vi "visa_write.vi"() -> ()   [LabVIEW 2016]
uses:
  <vilib>/Instr/_visa.llb/VISA Configure Serial Port (Instr).vi
panel:
  in  "停止":bool
  out "写入缓冲区":string
  out "输出数组":i32[](array[numeric])
  in  "目标位置":i32[](array[numeric])
  in  "当前位置":i32[](array[numeric])
  in  "串口配置":T1={"波特率"=115200, "奇偶校验位"=0, "停止位"=10, "流控制"=0, "数据位"=8} {"数据位" items=["8"=8]; "流控制" items=["无"=0, "XON/XOFF"=1, "RTS/CTS"=2, "DTR/DSR"=4]; "停止位" items=["1.0"=10, "2.0"=15, "3.0"=20]; "奇偶校验位" items=["None"]; "波特率" items=["115200"=115200]}
  in  "VISA资源名称":refnum<visa-resource-name>
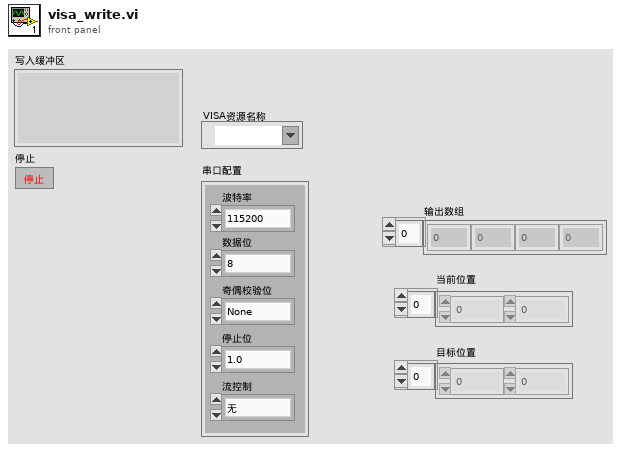
[diagram p1: front panel]
types:
  T1 = cluster{"波特率":u32, "奇偶校验位":u16, "停止位":u16, "流控制":u16, "数据位":u32}
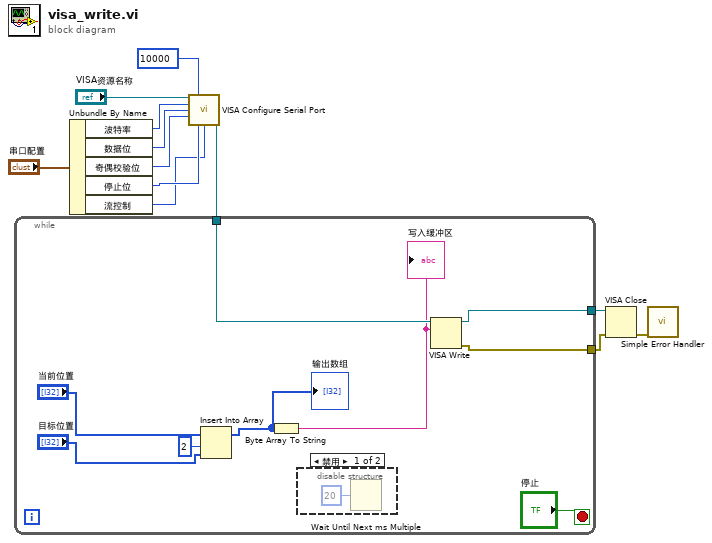
[diagram p0: block diagram]
diagram:
  n1 = Unbundle By Name("串口配置") -> ("波特率"=w10:u32, "数据位"=w9:u32, "奇偶校验位"=w8:u16, "停止位"=w7:u16, "流控制"=w6:u16)
  n2 = call-poly "VISA Configure Serial Port"("VISA resource name"="VISA资源名称", "timeout (10sec)"=u32 10000, "baud rate (9600)"=w10, "data bits (8)"=w9, "parity (0:none)"=w8, "stop bits (10: 1 bit)"=w7, "flow control (0:none)"=w6) -> ("VISA resource name out"=w5:refnum<visa-resource-name>)  [unwired: 7 in, 1 out]
  n3 = while {
    tunnel: w5 -> [w21]
    tunnel: [w14] -> w2
    tunnel: [w13] -> w1
    stop <- "停止" stop-if-true
    n4 = Insert Into Array(array="当前位置", index=2 ("索引"), new element="目标位置") -> (w15:i32[])
    "输出数组" <- w15
    n5 = Byte Array To String ("字节数组至字符串转换")(unsigned byte array=w15) -> (string=w20:string)
    "写入缓冲区" <- w20
    n6 = disable-structure shown="禁用" {
      frame Disabled {
        n7 = Wait Until Next ms Multiple(millisecond multiple=u32 20 ("毫秒倍数")) -> ()  [unwired: 1 out]
      }
      frame Enabled {
      }
    }
    n8 = VISA Write(VISA resource name=w21, write buffer=w20) -> (VISA resource name out=w14:refnum<visa-resource-name>, error out=w13:errorcluster)  [unwired: 1 in, 1 out]
  }
  n9 = VISA Close(VISA resource name=w2, error in (no error)=w1) -> (error out=w3:errorcluster)
  n10 = call <vilib>:"Simple Error Handler.vi"("error in (no error)"=w3) -> ()  [unwired: 4 in, 5 out]
